vi "Feedforward.vi"(4 "Final Weights":dbl[](array[numeric]), 5 "Function Final Layer":u16(ring) items=["Siqmoid", "Linear", "Sign"], 6 "Hidden Weights":dbl[][](array[numeric]), 7 "Inputs":dbl[](array[numeric]), 8 "Num Hidden Layer":i32, 9 "Function Hidden Layer":u16(ring) items=["Siqmoid", "Linear", "Sign"]) -> (0 "Function Hidden Layer 2":u16, 1 "Hidden Outputs":dbl[](array[numeric]), 2 "Output":dbl, 3 "Function Final Layer 2":u16)   [LabVIEW 2009]
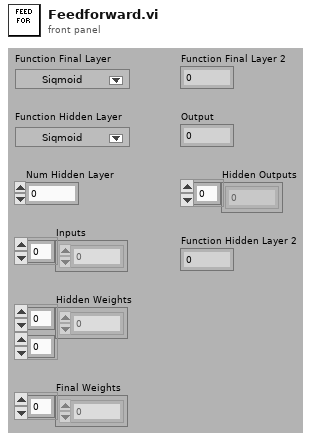
[diagram p1: front panel]
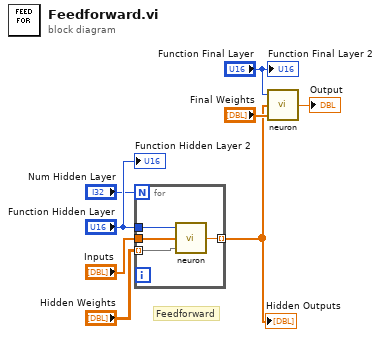
[diagram p0: block diagram]
diagram:
  # "Feedforward"
  n1 = for {
    N: "Num Hidden Layer" -> [_]
    tunnel: "Function Hidden Layer" -> [w12]
    tunnel: [w11] -> w4 mode=indexing
    tunnel: "Inputs" -> [w10]
    tunnel: "Hidden Weights" -> [w9] mode=indexing
    n2 = call "neuron.vi"("Weights"=w9, "Inputs"=w10, "Function"=w12) -> ("Output"=w11:dbl)
  }
  "Hidden Outputs" <- w4
  n3 = call "neuron.vi"("Weights"="Final Weights", "Inputs"=w4, "Function"="Function Final Layer") -> ("Output"=→"Output":dbl)
  "Function Hidden Layer 2" <- "Function Hidden Layer"
  "Function Final Layer 2" <- "Function Final Layer"
